vi "temperature.vi"() -> ()   [LabVIEW 2016]
panel:
  in  "stop":bool
  in  "Numeric":dbl
  out "Temperature (Deg F)":dbl(slide) scale=0.0..200.0
  out "Reading (Deg C)":dbl
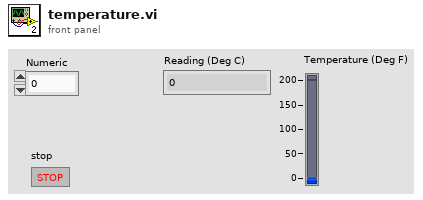
[diagram p1: front panel]
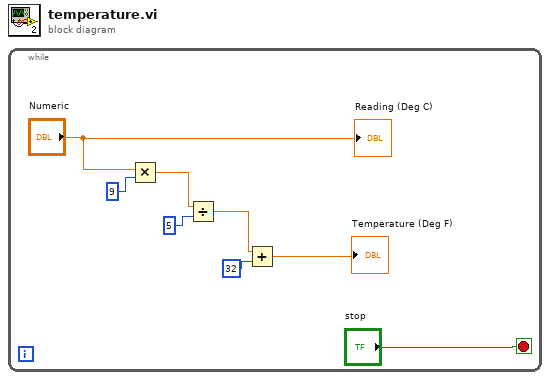
[diagram p0: block diagram]
diagram:
  n1 = while {
    stop <- "stop" stop-if-true
    n2 = Multiply(x="Numeric", y=9) -> (x*y=w5:dbl)
    n3 = Divide(x=w5, y=5) -> (x/y=w4:dbl)
    n4 = Add(x=w4, y=32) -> (x+y=→"Temperature (Deg F)":dbl)
    "Reading (Deg C)" <- "Numeric"
  }
